vi "New Human.vi"(8 "error in (no error)":errorcluster, 11 "Board Refnum":refnum<vi>) -> (0 "error out":errorcluster, 3 "Human out":refnum<class "Human.lvclass">)   [LabVIEW 2020, in "Reversi.lvlib" / "Human.lvclass"]
uses:
  Human.lvclass
  Space Ring.ctl
  Reversi.lvclass
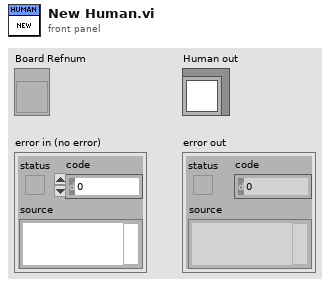
[diagram p1: front panel]
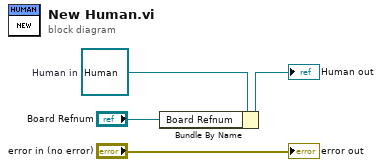
[diagram p0: block diagram]
diagram:
  w2 = refnum<class "Human.lvclass"> refnum  # Human in
  n1 = Bundle By Name(cluster=w2, "Board Refnum"="Board Refnum") -> (→"Human out":refnum<class "Human.lvclass">)
  "error out" <- "error in (no error)"
